vi "FGV_single cycle timestamps sequence.vi"(7 "ROI Dwell time (us)":dbl=4.0 min=0.05 max=20.0 step=0.05, 9 "Function":enum16{"Read", "Write", "Load", "Save"}(ring), 10 "Experiment folder path":path, 11 "Time-stamps (us) in":dbl[](array[numeric])) -> (1 "Funct Acq cycle length (us)":dbl, 3 "Single funct.acq cycle time-stamps (us)":dbl[](array[numeric]))   [LabVIEW 2020]
panel:
  out "all rows":dbl[][](array[numeric]) format="%0.3f"
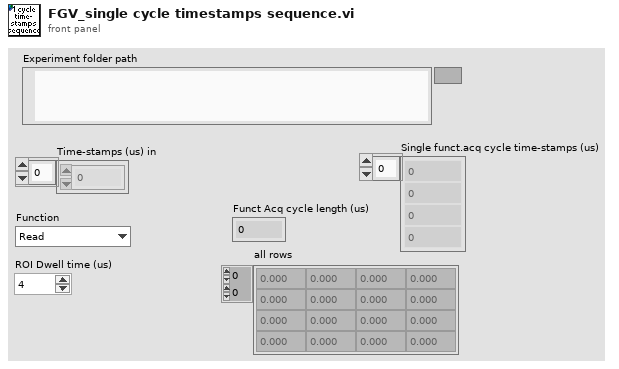
[diagram p1: front panel]
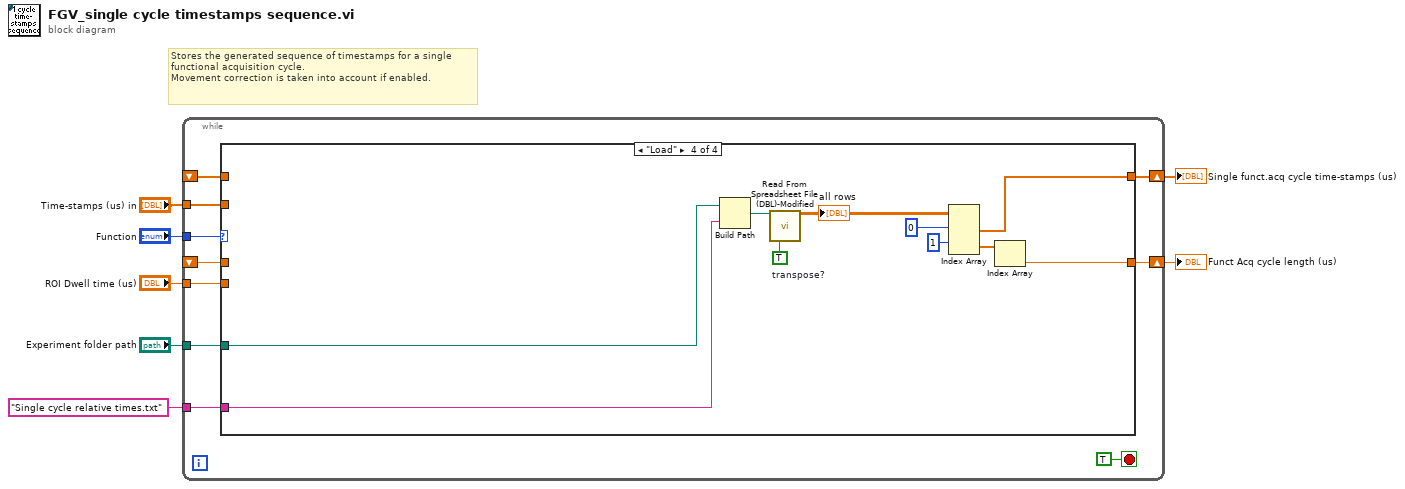
[diagram p0: block diagram]
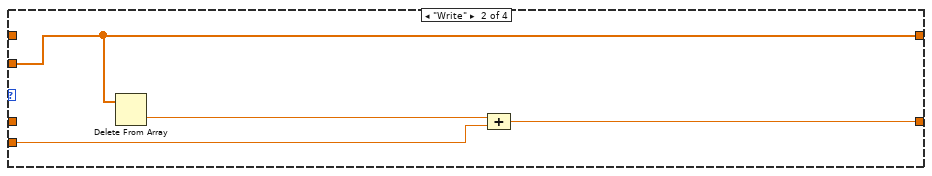
[diagram p3: hidden frame]
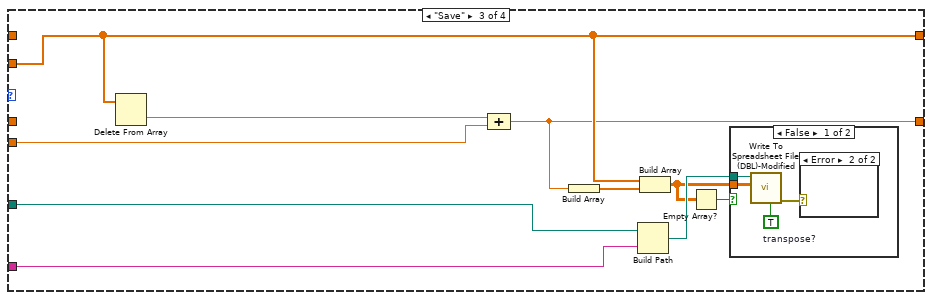
[diagram p4: hidden frame]
diagram:
  # "Stores the generated sequence of timestamps for a single functional acquisition cycle.\nMovement correction is taken into account if enabled."
  n1 = while {
    shift-right: [w15] -> w7
    shift-left: _ -> [w14]
    tunnel: "Time-stamps (us) in" -> [w16]
    tunnel: "Function" -> [w13]
    tunnel: "ROI Dwell time (us)" -> [w12]
    shift-right: [w11] -> w3
    shift-left: _ -> [w10]
    tunnel: "Single cycle relative times.txt" ("name or relative path") -> [w9]
    tunnel: "Experiment folder path" -> [w8]
    stop <- TRUE stop-if-true
    n2 = case shown="\"Load\"" w13 {
      tunnel: w16 -> [_ w20 w29 _]
      tunnel: [w19 w20 w29 w46] -> w15
      tunnel: w14 -> [w19 _ _ _]
      tunnel: w12 -> [_ w22 w32 _]
      tunnel: [w18 w21 w28 w43] -> w11
      tunnel: w10 -> [w18 _ _ _]
      tunnel: w9 -> [_ _ w27 w42]
      tunnel: w8 -> [_ _ w26 w41]
      frame "Read", Default {
      }
      frame "Write" {
        n3 = Delete From Array(array=w20) -> (deleted portion=w23:dbl)  [unwired: 2 in, 1 out]
        n4 = Compound Arithmetic op=ADD(w23, w22) -> (w21:dbl)
      }
      frame "Save" {
        n5 = Delete From Array(array=w29) -> (deleted portion=w33:dbl)  [unwired: 2 in, 1 out]
        n6 = Compound Arithmetic op=ADD(w33, w32) -> (w28:dbl)
        n7 = Build Array(w28) -> (w30:dbl[])
        n8 = Build Path(base path=w26, name or relative path=w27) -> (appended path=w31:path)
        n9 = Build Array(w29, w30) -> (w24:dbl[][])
        n10 = Empty Array?(array=w24) -> (empty?=w25:bool)
        n11 = case shown="False" w25 {
          tunnel: w24 -> [w37 _]
          tunnel: w31 -> [w36 _]
          frame False {
            w35 = TRUE  # transpose?
            n12 = call "Write To Spreadsheet File (DBL)-Modified.vi"("transpose? (no:F)"=w35, "2D data"=w37, "file path (dialog if empty)"=w36) -> ("error out"=w34:errorcluster)  [unwired: 7 in, 1 out]
            n13 = case shown="Error" w34 {
              frame No Error {
              }
              frame Error {
              }
            }
          }
          frame True {
          }
        }
      }
      frame "Load" {
        w39 = TRUE  # transpose?
        n14 = Build Path(base path=w41, name or relative path=w42) -> (appended path=w40:path)
        n15 = call "Read From Spreadsheet File (DBL)-Modified.vi"("file path (dialog if empty)"=w40, "transpose (no:F)"=w39) -> ("all rows"=w38:dbl[][])  [unwired: 8 in, 5 out]
        "all rows" <- w38
        n16 = Index Array(array=w38, index (row) #1=0 ("index (row)"), index (row) #2=1 ("index (row)")) -> (element #1=w46:dbl[], element #2=w44:dbl[])  [unwired: 2 in]
        n17 = Index Array(array=w44) -> (element=w43:dbl)  [unwired: 1 in]
      }
    }
  }
  "Single funct.acq cycle time-stamps (us)" <- w7
  "Funct Acq cycle length (us)" <- w3
